vi "Point_Create_double.vi"(8 "Error In":errorcluster, 10 "Tag":string, 11 "Map":T1) -> (0 "Error Out":errorcluster, 3 "Map Out":T1)   [LabVIEW 2017, in "PointValueMap.lvlib"]
doc: "Creates a new map point with a specified name but without a value."
uses:
  <vilib>/addons/PointValueMap/PointValueMap.lvlib
  <vilib>/addons/PointValueMap/controls/PointMap.ctl
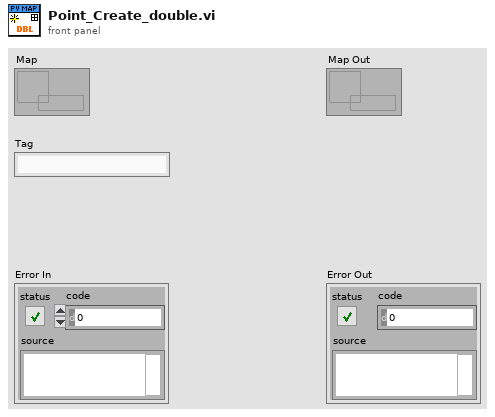
[diagram p1: front panel]
types:
  T1 = typedef "PointValueMap.lvlib/PointMap.ctl" = refnum<data-value>
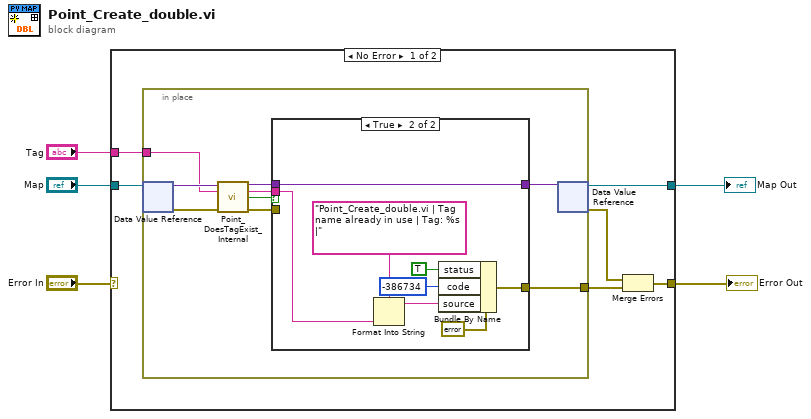
[diagram p0: block diagram]
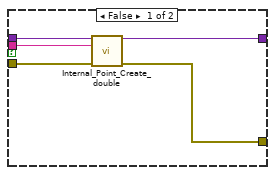
[diagram p2: hidden frame]
diagram:
  n1 = case shown="No Error" "Error In" {
    selector: "Error In" -> [_ w35]
    tunnel: "Map" -> [w11 w34]
    tunnel: "Tag" -> [w10 _]
    tunnel: [w7 w35] -> w4
    tunnel: [w6 w34] -> w1
    frame No Error {
      n2 = in-place {
        in-place-border: w10 -> [w14]
        in-place-border: [w19] -> w8
        n3 = in-place-dvr #1(w11) -> (w18:variant, w16:errorcluster)
        n4 = call <vilib>:"Point_DoesTagExist_Internal.vi"("Map"=w18, "Tag"=w14, "Error In"=w16) -> ("Map Out"=w17:variant, "Tag Out"=w12:string, "Tag Exists"=w13:bool, "Error Out"=w15:errorcluster)  [unwired: 7 in, 2 out]
        n5 = case shown="True" w13 {
          tunnel: [w25 w33] -> w20
          tunnel: [w24 w27] -> w19
          tunnel: w17 -> [w22 w33]
          tunnel: w15 -> [w23 _]
          tunnel: w12 -> [w21 w26]
          frame False {
            n6 = call <vilib>:"Internal_Point_Create_double.vi"("Internal Map (variant)"=w22, "Tag Name"=w21, "error in (no error)"=w23) -> ("Internal Map Out (variant)"=w25:variant, "error out"=w24:errorcluster)  [unwired: 8 in, 3 out]
          }
          frame True {
            n7 = Format Into String(format string="Point_Create_double.vi | Tag name already in use | Tag: %s |" ("source"), w26) -> (resulting string=w29:string)  [unwired: 2 in, 1 out]
            n8 = Bundle By Name(cluster=errorcluster {"status"=FALSE, "code"=0, "source"=""} ("Error Out"), "status"=TRUE, "code"=-386734, "source"=w29) -> (w27:errorcluster)
          }
        }
        n9 = in-place-dvr #1(w20) -> (w6:T1, w9:errorcluster)
      }
      n10 = Merge Errors(w9, w8) -> (w7:errorcluster)
    }
    frame Error {
    }
  }
  "Error Out" <- w4
  "Map Out" <- w1
